vi "LoadFGV.vi"(8 "error in":errorcluster) -> (0 "error out":errorcluster)   [LabVIEW 2021]
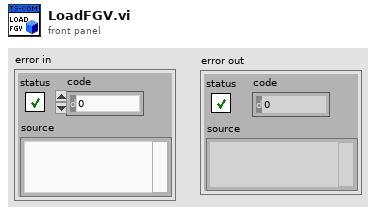
[diagram p1: front panel]
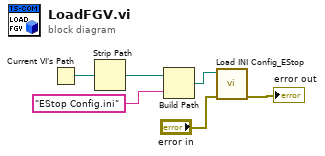
[diagram p0: block diagram]
diagram:
  n1 = Current VI's Path() -> (path=w2:path)
  n2 = Strip Path(path=w2) -> (stripped path=w1:path)  [unwired: 1 out]
  n3 = Build Path(base path=w1, name or relative path="EStop Config.ini") -> (appended path=w6:path)
  n4 = call "Load INI Config_EStop.vi"("error in"="error in", "configuration file path"=w6) -> ("error out"=→"error out":errorcluster)  [unwired: 9 in]
